vi "Group_Get_Name.vi"(8 "error in (no error)":errorcluster, 11 "Group in":refnum<class "Group.lvclass">) -> (0 "error out":errorcluster, 2 "Name":string, 3 "Group out":refnum<class "Group.lvclass">)   [LabVIEW 2023, in "Group.lvclass"]
doc: "Gets the name of the group."
uses:
  Group.lvclass
  Group.lvclass/Group.ctl
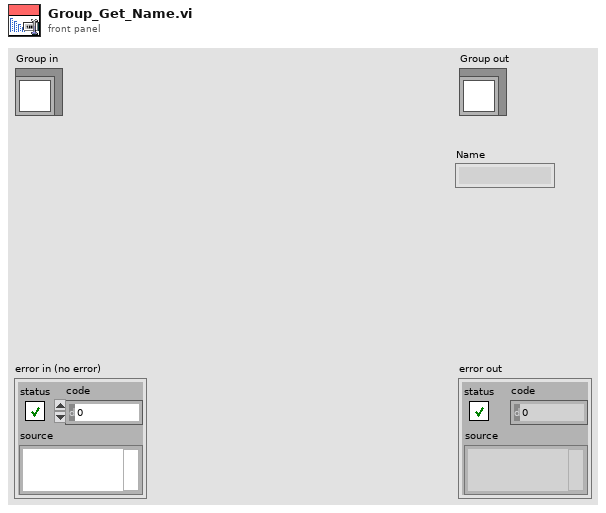
[diagram p1: front panel]
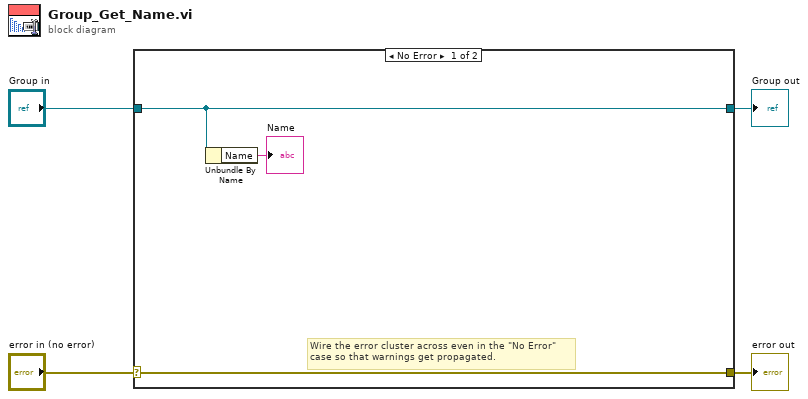
[diagram p0: block diagram]
diagram:
  n1 = case shown="No Error" "error in (no error)" {
    selector: "error in (no error)" -> [w7 w9]
    tunnel: [w7 w9] -> w3
    tunnel: [w6 w8] -> w1
    tunnel: "Group in" -> [w6 w8]
    frame No Error {
      # "Wire the error cluster across even in the \"No Error\"\ncase so that warnings get propagated."
      n2 = Unbundle By Name(w6) -> ("Name"=→"Name":string)
    }
    frame Error {
    }
  }
  "error out" <- w3
  "Group out" <- w1
